vi "Configure Power Supply Rejection Ratio Analysis (Basic).vi"(6 "Output Channel (1: Channel 2)":i32(ring)=1 items=["Channel 1", "Channel 2", "Channel 3", "Channel 4"], 7 "Input Channel (0: Channel 1)":i32(ring) items=["Channel 1", "Channel 2", "Channel 3", "Channel 4"], 8 "error in (no error)":errorcluster, 9 "Trace (1: Gain)":i32(ring)=1 items=["None", "Gain"], 10 "Point Number (10: 10)":i32(ring)=10 items=["10"=10, "20"=20, "30"=30, "40"=40, "50"=50, "60"=60, "70"=70, "80"=80, "90"=90, "100"=100], 11 "VISA resource name":refnum<visa-resource-name>) -> (0 "error out":errorcluster, 3 "VISA resource name out":refnum<visa-resource-name>)   [LabVIEW 2015, in "Agilent 2000 3000 X-Series.lvlib"]
doc: "Configures the basic setting for power supply rejection ratio (PSRR) power analysis.\n\n<b>Note:</b>\n - This VI is applicable for 3000T,3000G, 4000, 6000 X-Series."
uses:
  Agilent 2000 3000 X-Series.lvlib
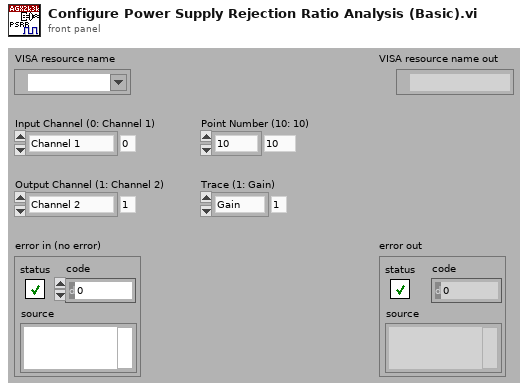
[diagram p1: front panel]
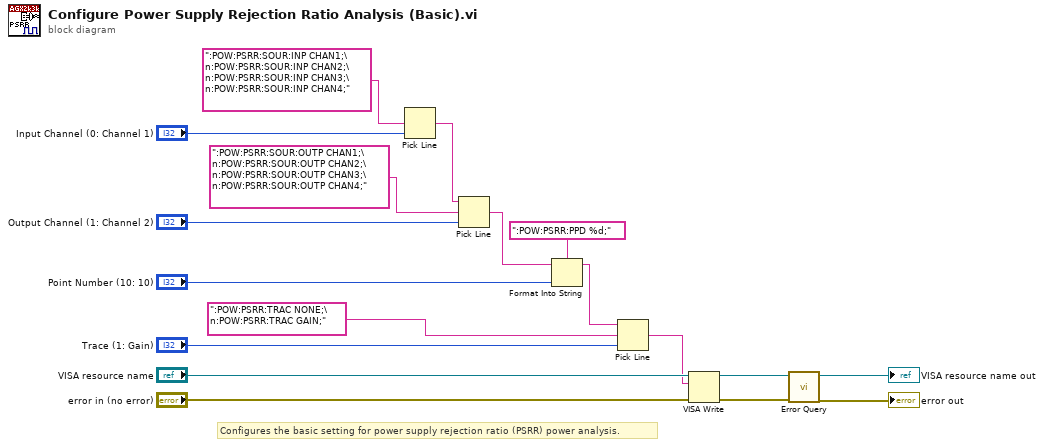
[diagram p0: block diagram]
diagram:
  # "Configures the basic setting for power supply rejection ratio (PSRR) power analysis."
  n1 = Pick Line(multi-line string=":POW:PSRR:SOUR:INP CHAN1;\n:POW:PSRR:SOUR:INP CHAN2;\n:POW:PSRR:SOUR:INP CHAN3;\n:POW:PSRR:SOUR:INP CHAN4;", line index="Input Channel (0: Channel 1)") -> (output string=w5:string)  [unwired: 1 in]
  n2 = Pick Line(string ("")=w5, multi-line string=":POW:PSRR:SOUR:OUTP CHAN1;\n:POW:PSRR:SOUR:OUTP CHAN2;\n:POW:PSRR:SOUR:OUTP CHAN3;\n:POW:PSRR:SOUR:OUTP CHAN4;", line index="Output Channel (1: Channel 2)") -> (output string=w4:string)
  n3 = Format Into String(format string=":POW:PSRR:PPD %d;", initial string=w4, "Point Number (10: 10)") -> (resulting string=w3:string)  [unwired: 1 in, 1 out]
  n4 = Pick Line(string ("")=w3, multi-line string=":POW:PSRR:TRAC NONE;\n:POW:PSRR:TRAC GAIN;", line index="Trace (1: Gain)") -> (output string=w2:string)
  n5 = VISA Write(VISA resource name="VISA resource name", write buffer=w2, error in (no error)="error in (no error)") -> (VISA resource name out=w9:refnum<visa-resource-name>, error out=w8:errorcluster)  [unwired: 1 out]
  n6 = call "Error Query.vi"("error in (no error)"=w8, "VISA resource name"=w9) -> ("error out"=→"error out":errorcluster, "VISA resource name out"=→"VISA resource name out":refnum<visa-resource-name>)  [unwired: 6 in, 2 out]
